vi "get_config_cluster.vi"(8 "error in (no error)":errorcluster, 11 "SignalWriterDL090202DAQmx in":refnum<class "SignalWriterMM140725DAQmx.lvclass">) -> (0 "error out":errorcluster, 2 "config cluster (variant)":variant, 3 "SignalWriterDL090202DAQmx out":refnum<class "SignalWriterMM140725DAQmx.lvclass">)   [LabVIEW 2010, in "SignalWriterMM140725DAQmx.lvclass"]
uses:
  SignalWriterMM140725DAQmx.lvclass
  SignalWriterMM140725DAQmx.lvclass/SignalWriterMM140725DAQmx.ctl
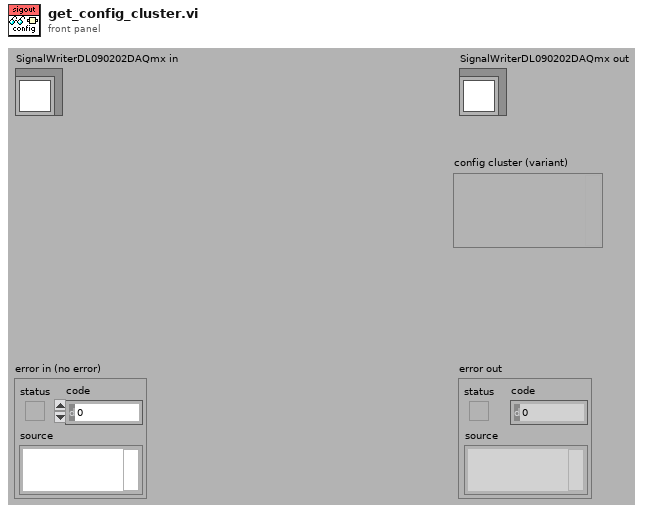
[diagram p1: front panel]
types:
  T1 = typedef "SignalWriterMM140725DAQmx.lvclass/config_data_cluster.ctl" = cluster{"physical channel":string, "timing source":string, "lag ":dbl[unit], "output type":string, "maximum output value":dbl, "minimum output value":dbl, "trigger line":string, "edge":T2, "counter":string}
  T2 = typedef "SignalWriterMM140725DAQmx.lvclass/trigger_edge_enum.ctl" = enum16{"rising", "falling"}
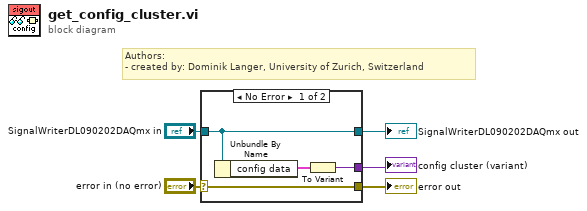
[diagram p0: block diagram]
diagram:
  # "Authors: \n- created by: Dominik Langer, University of Zurich, Switzerland"
  n1 = case shown="No Error" "error in (no error)" {
    selector: "error in (no error)" -> [w9 w11]
    tunnel: [w9 w11] -> w4
    tunnel: [w8 w10] -> w2
    tunnel: "SignalWriterDL090202DAQmx in" -> [w8 w10]
    tunnel: [w6 _] -> w1
    frame No Error {
      n2 = Unbundle By Name(w8) -> ("config data"=w7:T1)
      n3 = To Variant(anything=w7) -> (Variant=w6:variant)
    }
    frame Error {
    }
  }
  "error out" <- w4
  "SignalWriterDL090202DAQmx out" <- w2
  "config cluster (variant)" <- w1
